vi "Fetch Measurement (Read).vi"(8 "error in (no error)":errorcluster, 10 "Timeout (10000 ms)":u32=10000, 11 "VISA resource name":refnum<visa-resource-name>) -> (0 "error out":errorcluster, 1 "End of Data?":bool, 2 "Measurements":dbl[](array[numeric]), 3 "VISA resource name out":refnum<visa-resource-name>)   [LabVIEW 2020, in "Agilent 34401.lvlib"]
doc: "Fetches measurement from the instrument. This VI is to be used after \"READ?\" has been called. The VI will retrieve up to 10 data data points from the instrument's output buffer. This VI should be called repeatedly until End of Data? is True.\n\n<B>Note:</B>\n\nThis VI is called by <B>Fetch Measurement VI</B> in the following cases:\n(1) Model = 34401, Trigger Source = Immediate/External, and Math = Off/Output Buffer\n(2) Model = 34410/34411, Trigger Source = Immediate/External/Internal, and Math = On"
uses:
  <instrlib>/Agilent 34401/Agilent 34401.lvlib
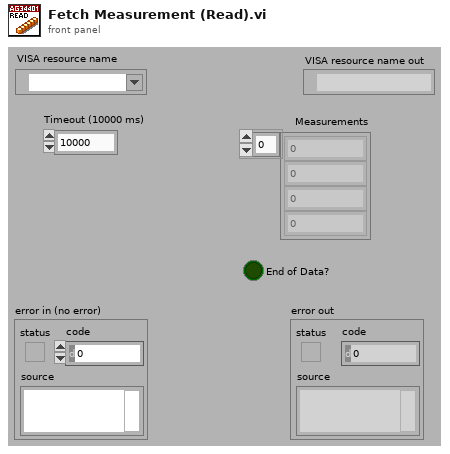
[diagram p1: front panel]
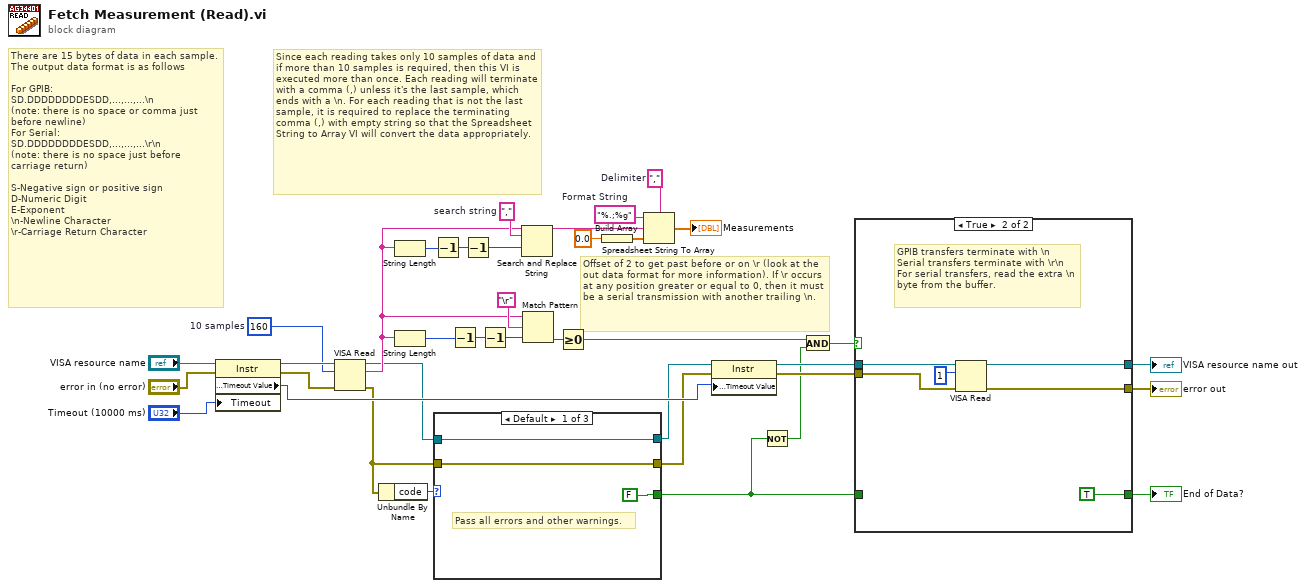
[diagram p0: block diagram]
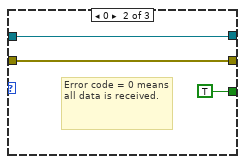
[diagram p2: hidden frame]
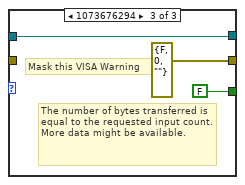
[diagram p3: hidden frame]
diagram:
  w26 = ","  # search string
  w36 = ","  # Delimiter
  w37 = "%.;%g"  # Format String
  w1 = u32 160  # 10 samples
  # "Offset of 2 to get past before or on \\r (look at the out data format for more information). If \\r occurs at any position greater or equal to 0, then it must be a serial transmission with another trailing \\n."
  # "Since each reading takes only 10 samples of data and if more than 10 samples is required, then this VI is executed more than once. Each reading will terminate with a comma (,) unless it's the last sample, which ends with a \\n. For each reading that is not the last sample, it is required to replace the terminating comma (,) with empty string so that the Spreadsheet String to Array VI will convert the data appropriately."
  # "There are 15 bytes of data in each sample. The output data format is as follows\n\nFor GPIB:\nSD.DDDDDDDDESDD,...,...,...\\n\n(note: there is no space or comma just before newline) \nFor Serial: \nSD.DDDDDDDDESDD,...,...,...\\r\\n\n(note: there is no space just before carriage return)\n\nS-Negative sign or positive sign\nD-Numeric Digit\nE-Exponent\n\\n-Newline Character\n\\r-Carriage Return Character"
  n1 = property on="Property Node" class="Instr"(reference="VISA resource name", error in="error in (no error)", "Timeout"="Timeout (10000 ms)") -> (reference out=w30:refnum<visa-resource-name>, error out=w29:errorcluster, "General Settings:Timeout Value"=w28:u32)
  n2 = VISA Read(VISA resource name=w30, byte count=w1, error in (no error)=w29) -> (VISA resource name out=w3:refnum<visa-resource-name>, read buffer=w16:string, error out=w12:errorcluster)  [unwired: 1 out]
  n3 = Unbundle By Name(w12) -> ("code"=w13:i32)
  n4 = String Length(string=w16) -> (length=w23:i32)
  n5 = String Length(string=w16) -> (length=w18:i32)
  n6 = Decrement(x=w23) -> (x-1=w24:i32)
  n7 = case shown="Default" w13 {
    tunnel: w12 -> [w40 w41 _]
    tunnel: [w40 w41 errorcluster {"status"=FALSE, "code"=0, "source"=""} ("error out")] -> w11
    tunnel: [FALSE TRUE FALSE] -> w7
    tunnel: w3 -> [w38 w42 w44]
    tunnel: [w38 w42 w44] -> w2
    frame Default {
      # "Pass all errors and other warnings."
    }
    frame 0 {
      # "Error code = 0 means all data is received."
    }
    frame 1073676294 {
      # "Mask this VISA Warning"
      # "The number of bytes transferred is equal to the requested input count. More data might be available."
    }
  }
  n8 = Decrement(x=w18) -> (x-1=w19:i32)
  n9 = Decrement(x=w24) -> (x-1=w22:i32)
  n10 = Decrement(x=w19) -> (x-1=w17:i32)
  n11 = Search and Replace String(input string=w16, search string=w26, offset=w22) -> (result string=w25:string)  [unwired: 5 in, 3 out]
  n12 = Match Pattern(string=w16, regular expression="\r" ("Carriage Return Constant"), offset (0)=w17) -> (offset past match=w20:i32)  [unwired: 3 out]
  n13 = Greater Or Equal To 0?(x=w20) -> (x >= 0?=w9:bool)
  n14 = Build Array(0.0) -> (w34:dbl[])
  n15 = Spreadsheet String To Array(delimiter (Tab)=w36, format string=w37, spreadsheet string=w25, array type (2D Dbl)=w34) -> (array=→"Measurements":dbl[])
  n16 = property on="Property Node" class="Instr"(reference=w2, error in=w11, "General Settings:Timeout Value"=w28) -> (reference out=w15:refnum<visa-resource-name>, error out=w14:errorcluster)
  n17 = Not(x=w7) -> (.not. x?=w8:bool)
  n18 = And(x=w9, y=w8) -> (x .and. y?=w10:bool)
  n19 = case shown="True" w10 {
    tunnel: w15 -> [w49 w55]
    tunnel: w14 -> [w48 w54]
    tunnel: [w49 w52] -> w4
    tunnel: [w48 w50] -> w5
    tunnel: w7 -> [w47 _]
    tunnel: [w47 TRUE] -> w6
    frame False {
      # "For GPIB transfers, error condition, or incomplete serial operations, pass VISA session, error cluster and previously determined End of Data Boolean."
    }
    frame True {
      # "GPIB transfers terminate with \\n\nSerial transfers terminate with \\r\\n\nFor serial transfers, read the extra \\n byte from the buffer."
      n20 = VISA Read(VISA resource name=w55, byte count=u32 1, error in (no error)=w54) -> (VISA resource name out=w52:refnum<visa-resource-name>, error out=w50:errorcluster)  [unwired: 2 out]
    }
  }
  "VISA resource name out" <- w4
  "error out" <- w5
  "End of Data?" <- w6
